vi "SpecAn BW Read.vi"(0 "VISA In":refnum<visa-resource-name>, 5 "Error In":errorcluster) -> (6 "Auto RBW (T: Enable)":bool=TRUE, 8 "Manual RBW":i32=3000000 format="%#.5p", 10 "Auto VBW (T: Enable)":bool=TRUE, 12 "Manual VBW":i32=3000001 format="%#.5p", 14 "VISA Out":refnum<visa-resource-name>, 19 "Error Out":errorcluster)   [LabVIEW 2015]
uses:
  Controls/FGV Action SpecAn Model.ctl
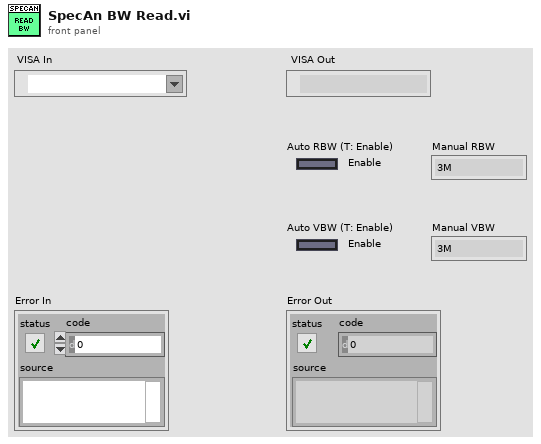
[diagram p1: front panel]
types:
  T1 = typedef "FGV Action SpecAn Model.ctl" = enum16{"Get", "Set"}
  T2 = typedef "SpecAn Model.ctl" = enum16{"E4440", "N9030"}
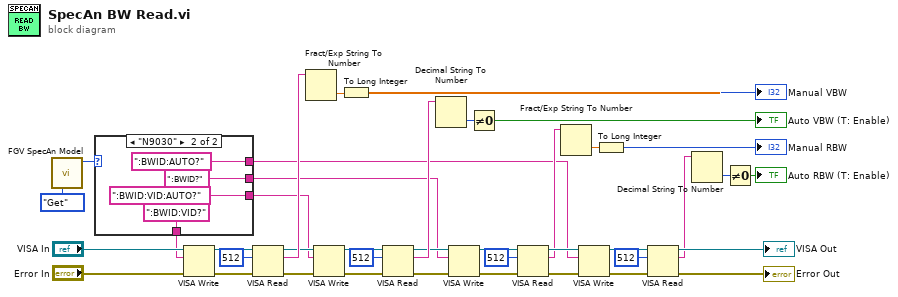
[diagram p0: block diagram]
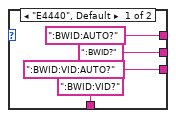
[diagram p2: hidden frame]
diagram:
  n1 = call "FGV SpecAn Model.vi"("Action"=FGV_Action_SpecAn_Model."Get") -> ("SA Model"=w37:T2)  [unwired: 6 in, 1 out]
  n2 = case shown="\"N9030\"" w37 {
    tunnel: [":BWID:VID?" ("format string") ":BWID:VID?" ("format string")] -> w32
    tunnel: [":BWID:VID:AUTO?" ("format string") ":BWID:VID:AUTO?" ("format string")] -> w23
    tunnel: [":BWID?" ("format string") ":BWID?" ("format string")] -> w5
    tunnel: [":BWID:AUTO?" ("format string") ":BWID:AUTO?" ("format string")] -> w4
    frame "E4440", Default {
    }
    frame "N9030" {
    }
  }
  n3 = VISA Write(VISA resource name="VISA In", write buffer=w32, error in (no error)="Error In") -> (VISA resource name out=w33:refnum<visa-resource-name>, error out=w34:errorcluster)  [unwired: 1 out]
  n4 = VISA Read(VISA resource name=w33, byte count=u32 512, error in (no error)=w34) -> (VISA resource name out=w25:refnum<visa-resource-name>, read buffer=w35:string, error out=w24:errorcluster)  [unwired: 1 out]
  n5 = Fract/Exp String To Number(string=w35) -> (number=w31:dbl)  [unwired: 3 in, 1 out]
  n6 = VISA Write(VISA resource name=w25, write buffer=w23, error in (no error)=w24) -> (VISA resource name out=w29:refnum<visa-resource-name>, error out=w28:errorcluster)  [unwired: 1 out]
  n7 = To Long Integer(number=w31) -> (32bit integer=→"Manual VBW":i32)
  n8 = VISA Read(VISA resource name=w29, byte count=u32 512, error in (no error)=w28) -> (VISA resource name out=w12:refnum<visa-resource-name>, read buffer=w27:string, error out=w11:errorcluster)  [unwired: 1 out]
  n9 = Decimal String To Number(string=w27) -> (number=w22:i32)  [unwired: 2 in, 1 out]
  n10 = VISA Write(VISA resource name=w12, write buffer=w5, error in (no error)=w11) -> (VISA resource name out=w15:refnum<visa-resource-name>, error out=w14:errorcluster)  [unwired: 1 out]
  n11 = Not Equal To 0?(x=w22) -> (x != 0?=→"Auto VBW (T: Enable)":bool)
  n12 = VISA Read(VISA resource name=w15, byte count=u32 512, error in (no error)=w14) -> (VISA resource name out=w19:refnum<visa-resource-name>, read buffer=w7:string, error out=w20:errorcluster)  [unwired: 1 out]
  n13 = Fract/Exp String To Number(string=w7) -> (number=w1:dbl)  [unwired: 3 in, 1 out]
  n14 = VISA Write(VISA resource name=w19, write buffer=w4, error in (no error)=w20) -> (VISA resource name out=w16:refnum<visa-resource-name>, error out=w17:errorcluster)  [unwired: 1 out]
  n15 = To Long Integer(number=w1) -> (32bit integer=→"Manual RBW":i32)
  n16 = VISA Read(VISA resource name=w16, byte count=u32 512, error in (no error)=w17) -> (VISA resource name out=→"VISA Out":refnum<visa-resource-name>, read buffer=w6:string, error out=→"Error Out":errorcluster)  [unwired: 1 out]
  n17 = Decimal String To Number(string=w6) -> (number=w8:i32)  [unwired: 2 in, 1 out]
  n18 = Not Equal To 0?(x=w8) -> (x != 0?=→"Auto RBW (T: Enable)":bool)
